vi "Enable Reference Group.vi"(11 "Ref Group":refnum<vi>[](array[refnum])) -> ()   [LabVIEW 2024]
uses:
  Enable.vi
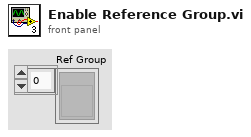
[diagram p1: front panel]
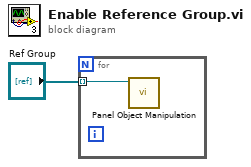
[diagram p0: block diagram]
diagram:
  n1 = for {
    tunnel: "Ref Group" -> [w2] mode=indexing
    n2 = call-poly "Panel Object Manipulation.vi"("Ctl Refnum"=w2) -> ()  [unwired: 10 in, 1 out]
  }
